vi "Separate Array Values.vi"(0 "输入数组":dbl[](array[numeric])=[6.0, 3.9, -5.8, 0.0, -2.6, -1.0, 2.2, -4.3]) -> (1 "正数数组":dbl[](array[numeric]), 2 "负数数组":dbl[](array[numeric]))   [LabVIEW 2012]
doc: "该VI可将包含正数和负数的数组分解为分别包含正数和负数的两个数组。\n\n条件自动索引用于区分正数和负数。"
panel:
  # "本VI可将输入数组拆分为两个分别包含正数和负数的一维数组。"
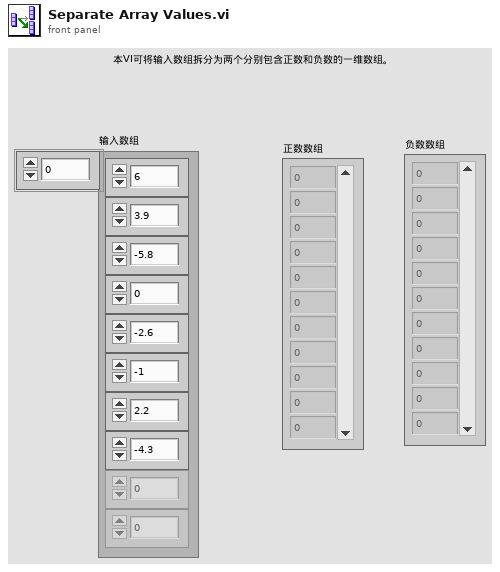
[diagram p1: front panel]
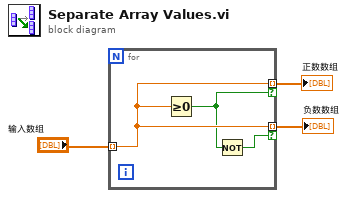
[diagram p0: block diagram]
diagram:
  n1 = for {
    tunnel: "输入数组" -> [w6] mode=indexing
    tunnel: [w6] -> w2 mode=indexing if=w5
    tunnel: [w6] -> w1 mode=indexing if=w4
    n2 = Greater Or Equal To 0? ("大于等于0？")(x=w6) -> (x >= 0?=w5:bool)
    n3 = Not ("非")(x=w5) -> (.not. x?=w4:bool)
  }
  "正数数组" <- w2
  "负数数组" <- w1
